vi "Get Turbo Valve Value.vi"(8 "error in (no error)":errorcluster, 11 "ILC PSV Open Loop Actuator Cylinder in":refnum<class "ILC PSV Open Loop Actuator Cylinder.lvclass">) -> (0 "error out":errorcluster, 2 "Value":dbl format="%.2f", 3 "ILC PSV Open Loop Actuator Cylinder out":refnum<class "ILC PSV Open Loop Actuator Cylinder.lvclass">)   [LabVIEW 2015, in "ILC PSV Open Loop Actuator Cylinder.lvclass"]
uses:
  ILC PSV Open Loop Actuator Cylinder.lvclass
  ILC Actuator Cylinder/ILC Actuator Cylinder.lvclass/ILC Actuator Cylinder.ctl
  ILC Actuator Cylinder/ILC Actuator Cylinder.lvclass
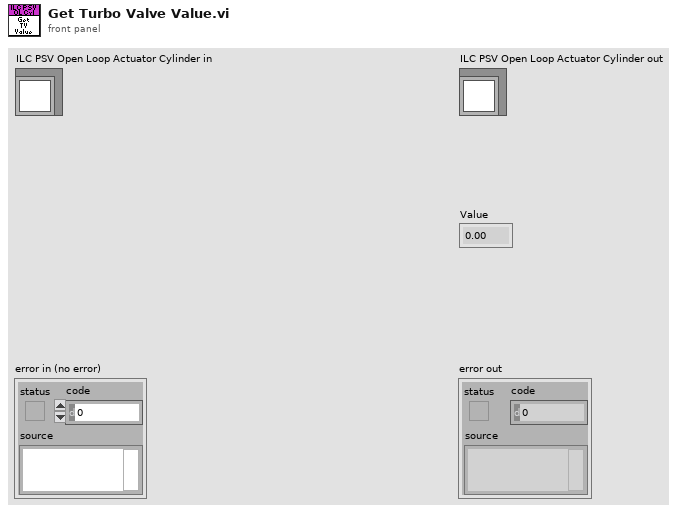
[diagram p1: front panel]
types:
  T1 = typedef "FAMT Typedefs.lvlib/Turbo Valve Settings.ctl" = cluster{"ROT Bias":u8, "Minimum Voltage":dbl, "Maximum Voltage":dbl, "Off Value":dbl}
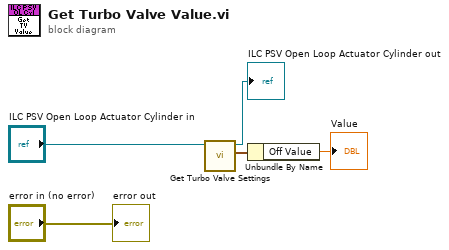
[diagram p0: block diagram]
diagram:
  n1 = call "Get Turbo Valve Settings.vi"("ILC Actuator Cylinder in"="ILC PSV Open Loop Actuator Cylinder in") -> ("Turbo Valve Settings"=w1:T1, "ILC Actuator Cylinder out"=→"ILC PSV Open Loop Actuator Cylinder out":refnum<class "ILC PSV Open Loop Actuator Cylinder.lvclass">)  [unwired: 9 in]
  n2 = Unbundle By Name(w1) -> ("Off Value"=→"Value":dbl)
  "error out" <- "error in (no error)"
